vi "main.vi"() -> ()   [LabVIEW 2018]
uses:
  <vilib>/NI/Modbus Library/API/Wrapper/Create TCP Slave.vi
  <vilib>/NI/Modbus Library/API/Slave/Modbus Slave.lvclass
  <vilib>/NI/Modbus Library/API/Wrapper/API Main.lvlib
panel:
  out "TCP Connection Count":u32
  in  "擦除曲线":bool
  in  "PC启动信号":bool
  in  "PC就绪":bool
  out "远程/本地控制布尔":bool
  out "XY图":cluster{i32[], sgl[]}[](graph)
  in  "远程/本地控制":bool
  out "远程/本地控制标题":string="远程/本地"
  out "当前档位":string="当前档位"
  in  "档位目标内容":string
  out "PCTOUTAC的当前档位":string="PCTOUTAC的当前档位"
  out "档位目标内容远程":string
  in  "档位目标内容本地":string
  out "档位目标":string="配方编号"
  out "UTACTOPC的目标档位":string="UTACTOPC的配方编号"
  in  "中英文":string(combo)
  in  "编辑设定参数":bool
  in  "编辑配方":bool
  in  "退出":bool
  out "设置":string="设置"
  in  "PC换挡不成功":bool
  in  "PC换挡到位":bool
  in  "PC正在换挡":bool
  in  "PC急停":bool
  in  "PC学习":bool
  in  "PC故障":bool
  in  "PC运行/停机":bool
  out "PCOUTAC的DI信号":string="PCTOUTAC的DI信号"
  in  "UTAC复位到原点":bool
  in  "UTAC故障复位":bool
  in  "UTAC急停":bool
  in  "UTAC故障":bool
  in  "UTAC运行/停机":bool
  out "UTACTOPC的DO信号":string="UTACTOPC的DO信号"
  in  "设置":bool
  in  "总测试次数文本":string
  in  "动作数量文本":string
  in  "备注文本":string
  in  "样品编号文本":string
  in  "零件编号文本":string
  in  "零件名称文本":string
  in  "项目编号文本":string
  out "总测试次数":string="总测试次数"
  out "动作数量":string="动作数量"
  out "备注":string="备注"
  out "样品编号":string="样品编号"
  out "零件编号":string="零件编号"
  out "零件名称":string="零件名称"
  out "项目编号":string="项目编号"
  out "项目信息":string="项目信息"
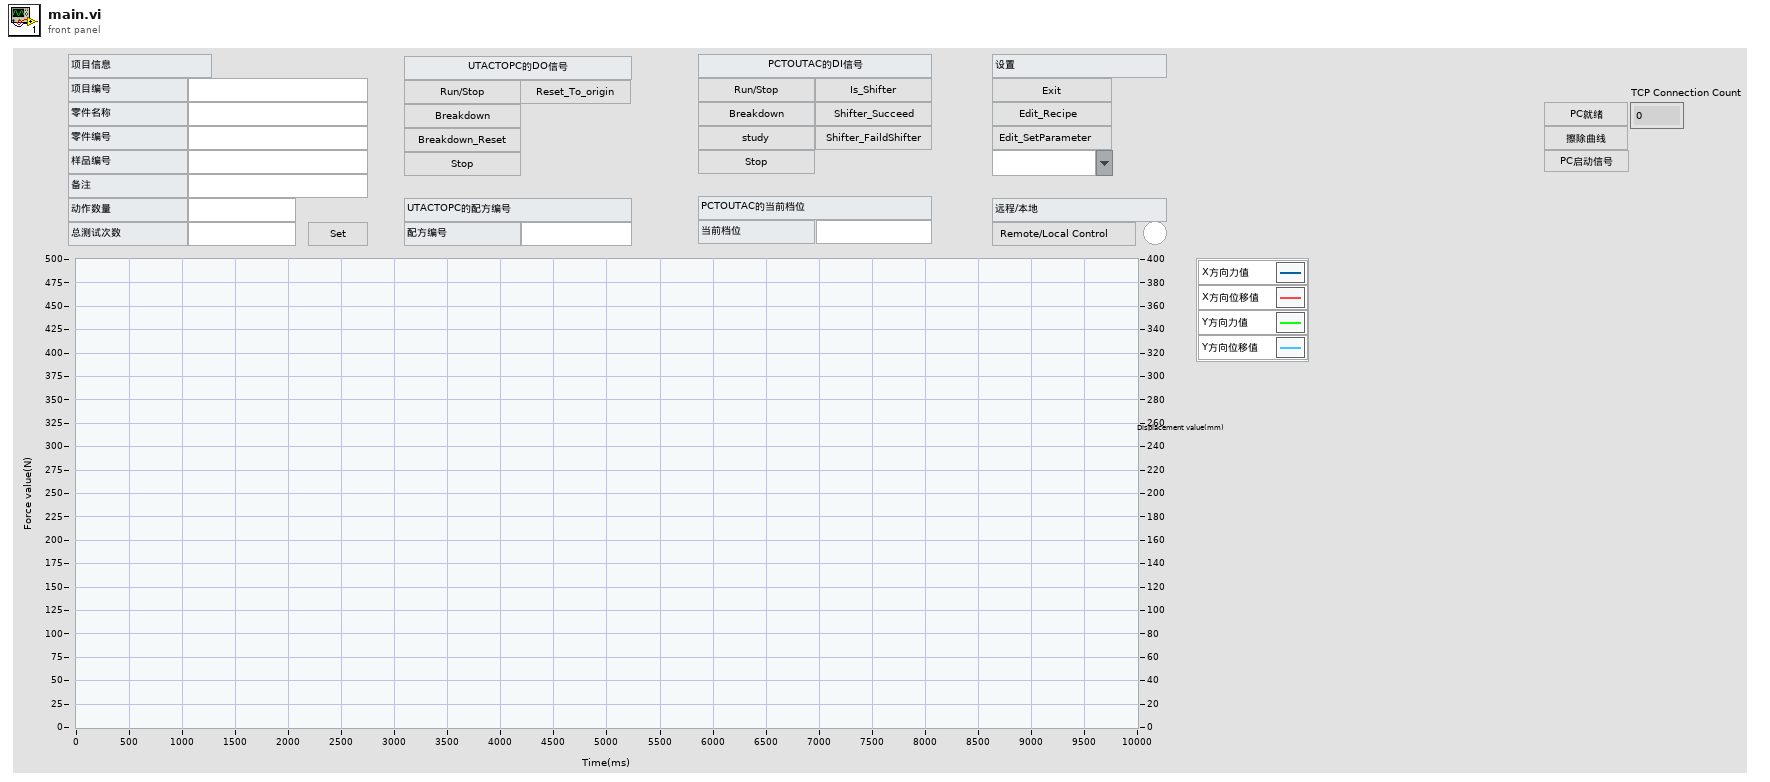
[diagram p1: front panel]
types:
  T1 = cluster{"主站IP":u32, "组号":u8, "帧号":u16, "时间戳":u64}
  T2 = cluster{"X方向力值":sgl, "Y方向力值":sgl, "X方向位移值":sgl, "Y方向位移值":sgl}
  T3 = cluster{"挡位N1所在序号":sgl, "挡位1所在序号":sgl, "挡位N1所在序号":sgl, "挡位2所在序号":sgl, "挡位N1所在序号":sgl, " 挡位N2所在序号":sgl, "挡位3所在序号":sgl, "挡位N2所在序号":sgl, "挡位4所在序号":sgl, " 挡位N2所在序号":sgl, "挡位N3所在序号":sgl, "挡位5所在序号":sgl, "挡位N3所在序号":sgl, "挡位6所在序号":sgl, "挡位N3所在序号":sgl, "挡位N4所在序号":sgl, " 挡位7所在序号":sgl, " 挡位N4所在序号":sgl, "挡位8所在序号":sgl, "挡位N4所在序号":sgl, " 挡位N5所在序号":sgl, "挡位9所在序号":sgl, "挡位N5所在序号":sgl, " 挡位10所在序号":sgl}
  T4 = cluster{"就绪":bool, "运行/停机":bool, "故障":bool, "学习":bool, "急停":bool, "正在换挡":bool, "换挡到位":bool, "换挡不成功":bool, "备用1":bool, "保存开始":bool, "等待下发任务":bool, "允许读取配方":bool, "开始采集数据":bool, "时间ON/OFF":bool, " 收到启动信号":bool, "结束采集信号":bool, "读配方参数ON/OFF":bool, "允许下发配方参数":bool}
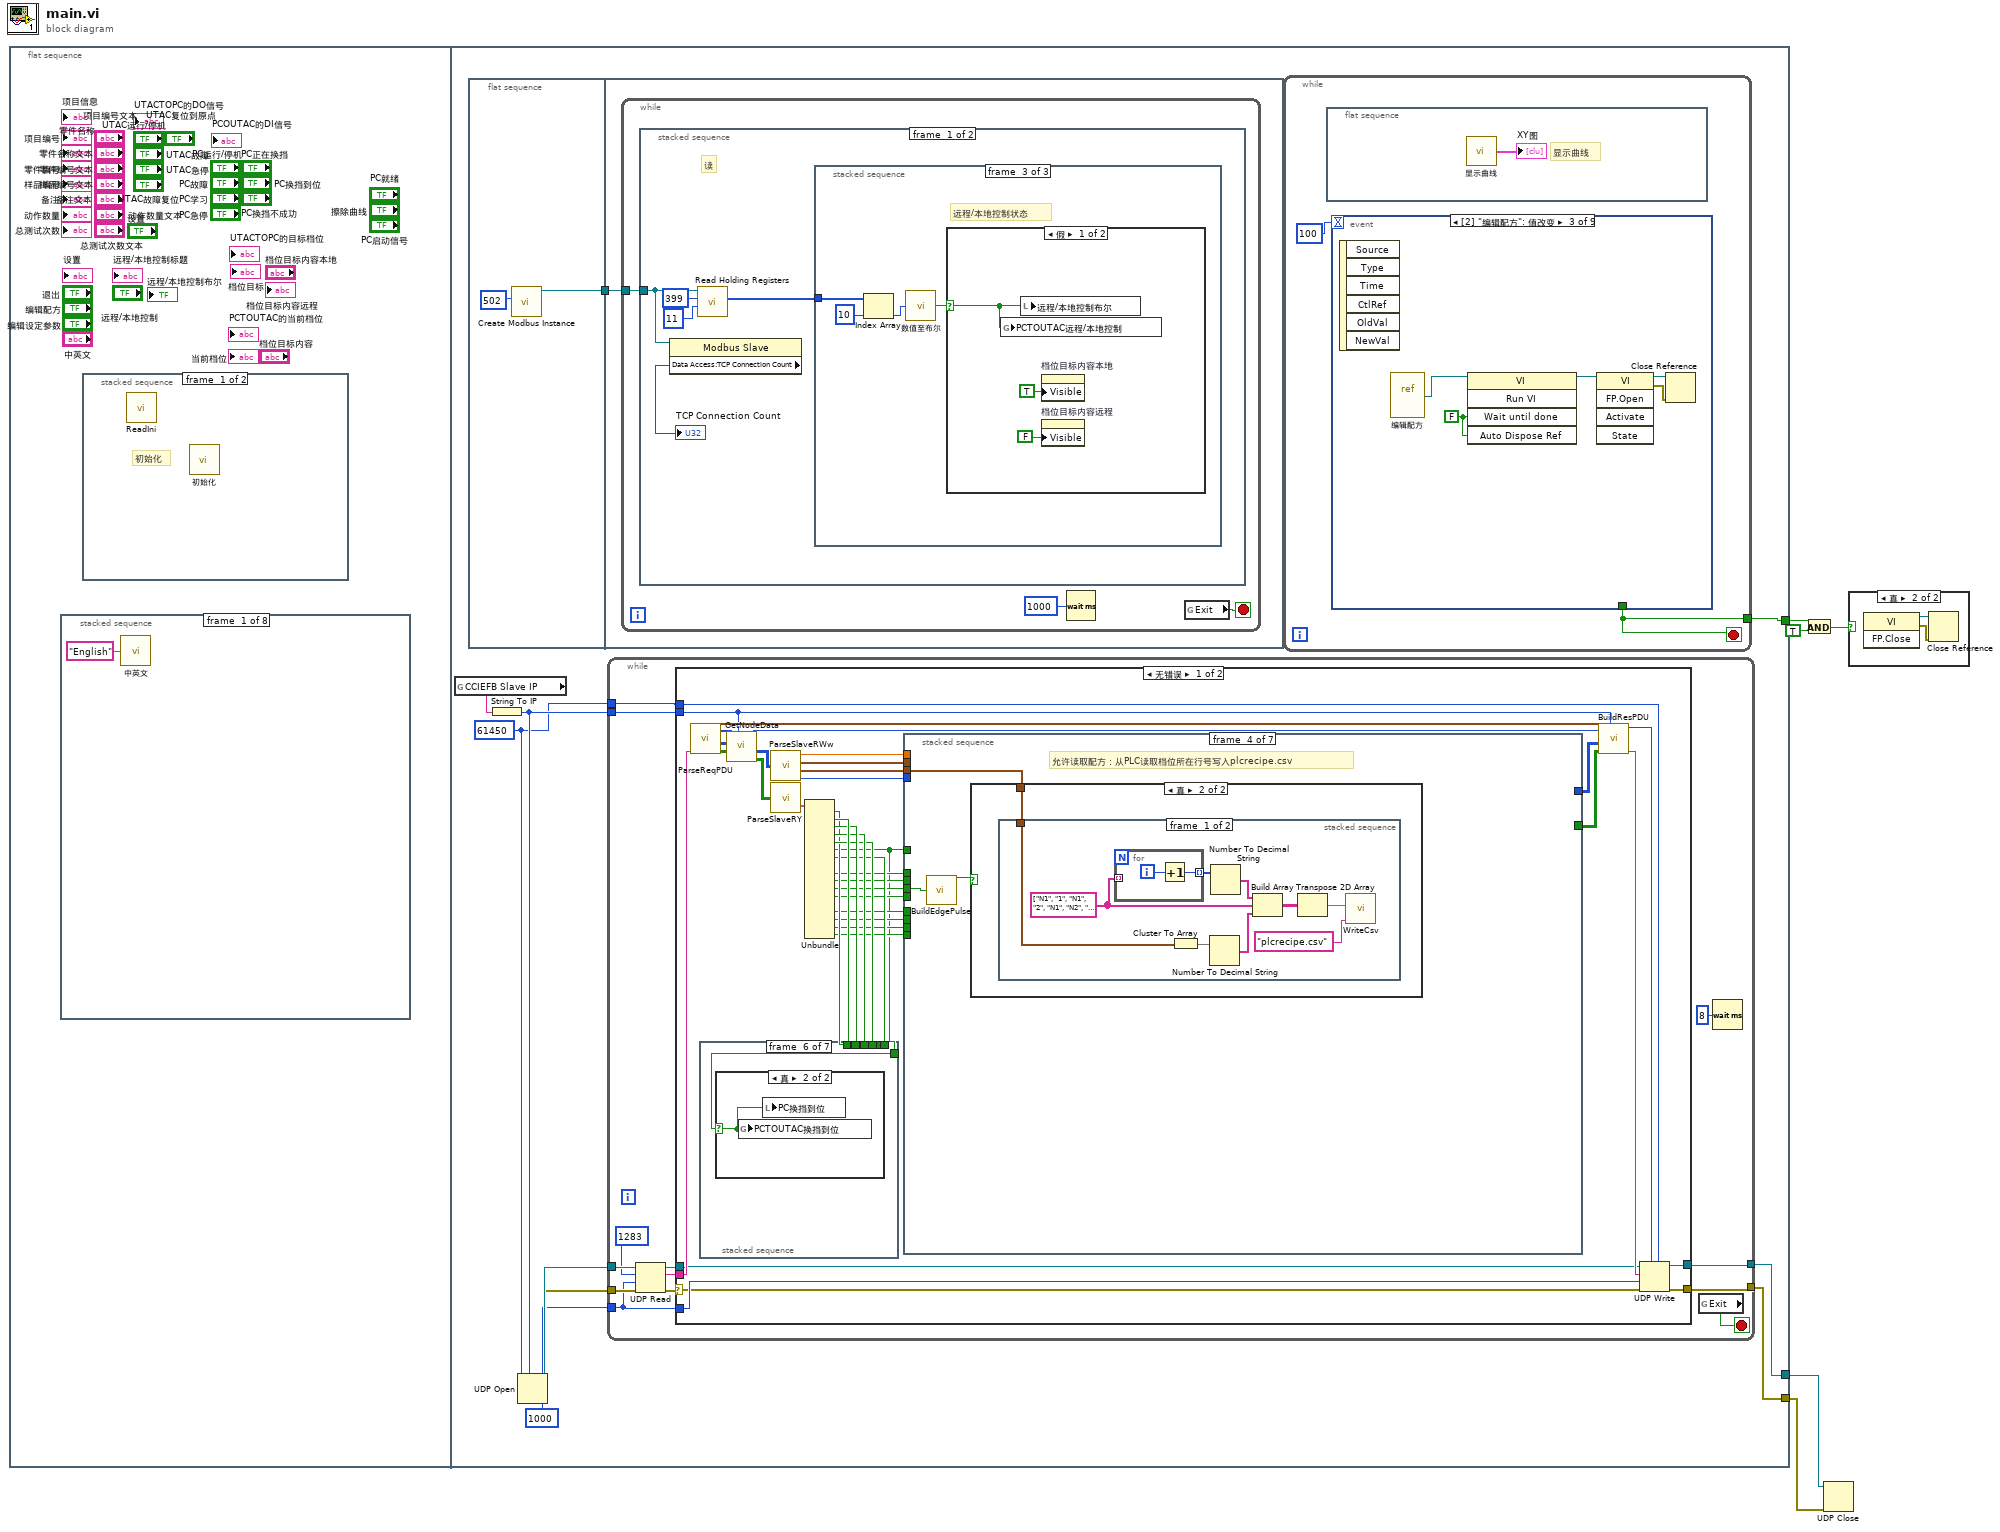
[diagram p0: block diagram]
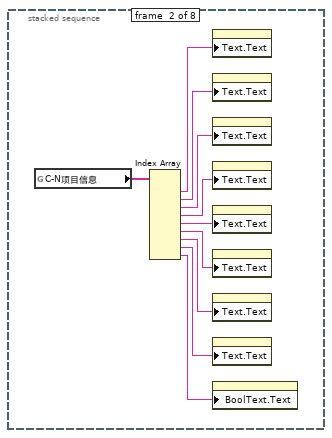
[diagram p3: hidden frame]
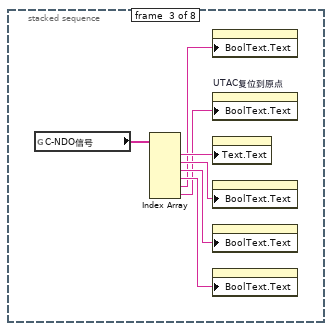
[diagram p4: hidden frame]
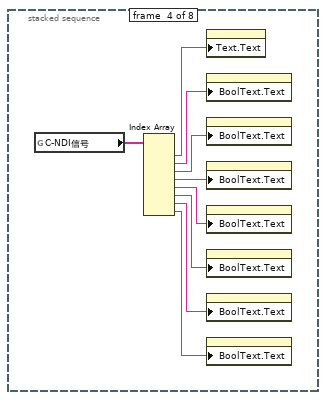
[diagram p5: hidden frame]
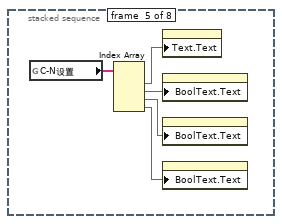
[diagram p6: hidden frame]
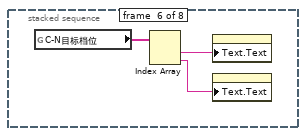
[diagram p7: hidden frame]
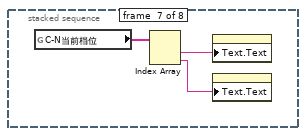
[diagram p8: hidden frame]
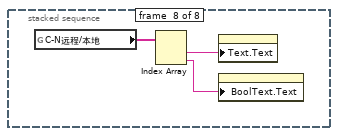
[diagram p9: hidden frame]
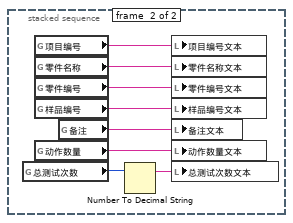
[diagram p10: hidden frame]
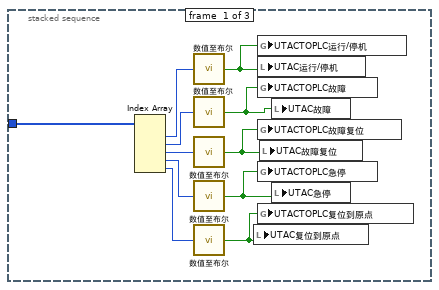
[diagram p11: hidden frame]
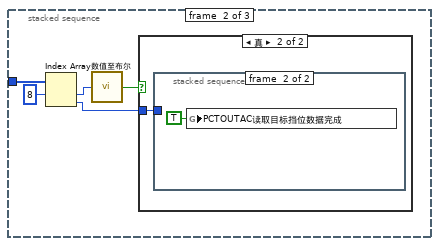
[diagram p12: hidden frame]
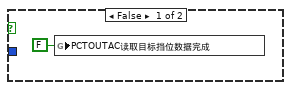
[diagram p13: hidden frame]
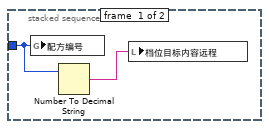
[diagram p14: hidden frame]
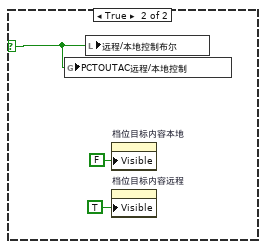
[diagram p15: hidden frame]
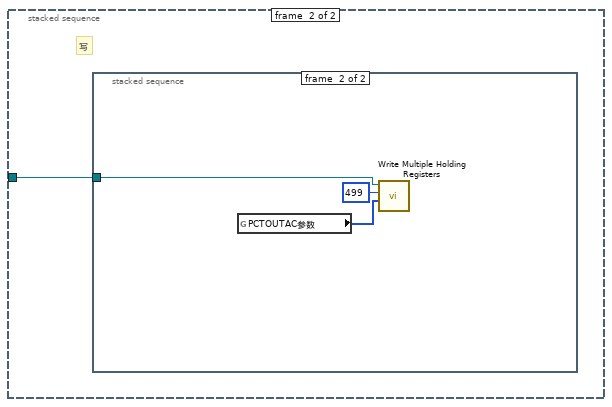
[diagram p16: hidden frame]
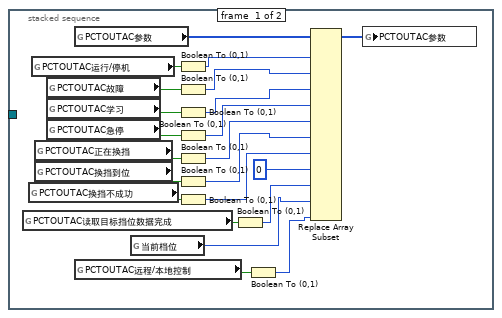
[diagram p17: hidden frame]
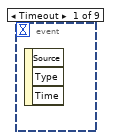
[diagram p18: hidden frame]
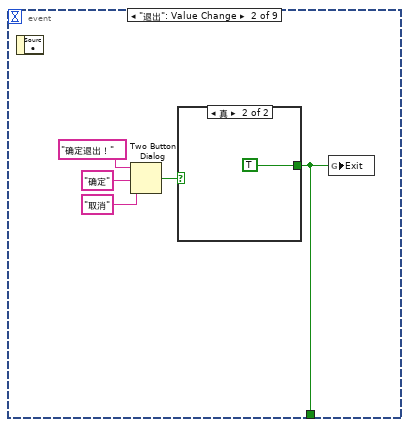
[diagram p19: hidden frame]
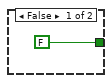
[diagram p20: hidden frame]
diagram:
  n1 = flat-sequence {
    tunnel: [w62] -> w5
    tunnel: [w61] -> w4
    tunnel: [w56] -> w3
    frame #0 {
      n2 = stacked-sequence {
        frame #0 {
          n3 = call "中英文.vi"("中英文"="English") -> ()  [unwired: 2 in]
        }
        frame #1 {
          n4 = global read "全局 1.vi" "C-N项目信息"() -> (w16:string[])
          n5 = Index Array(array=w16) -> (element #1=w15:string, element #2=w14:string, element #3=w13:string, element #4=w12:string, element #5=w11:string, element #6=w10:string, element #7=w9:string, element #8=w8:string, element #9=w7:string)  [unwired: 9 in]
          n6 = property on="项目信息" class="Str"("Text.Text"=w15) -> ()  [unwired: 2 in, 2 out]
          n7 = property on="项目编号" class="Str"("Text.Text"=w14) -> ()  [unwired: 2 in, 2 out]
          n8 = property on="零件名称" class="Str"("Text.Text"=w13) -> ()  [unwired: 2 in, 2 out]
          n9 = property on="零件编号" class="Str"("Text.Text"=w12) -> ()  [unwired: 2 in, 2 out]
          n10 = property on="样品编号" class="Str"("Text.Text"=w11) -> ()  [unwired: 2 in, 2 out]
          n11 = property on="备注" class="Str"("Text.Text"=w10) -> ()  [unwired: 2 in, 2 out]
          n12 = property on="动作数量" class="Str"("Text.Text"=w9) -> ()  [unwired: 2 in, 2 out]
          n13 = property on="总测试次数" class="Str"("Text.Text"=w8) -> ()  [unwired: 2 in, 2 out]
          n14 = property on="设置" class="Bool"("BoolText.Text"=w7) -> ()  [unwired: 2 in, 2 out]
        }
        frame #2 {
          n15 = global read "全局 1.vi" "C-NDO信号"() -> (w23:string[])
          n16 = Index Array(array=w23) -> (element #1=w22:string, element #2=w21:string, element #3=w20:string, element #4=w19:string, element #5=w18:string, element #6=w17:string)  [unwired: 6 in]
          n17 = property on="UTAC急停" class="Bool (严格)"("BoolText.Text"=w18) -> ()  [unwired: 2 in, 2 out]
          n18 = property on="UTAC复位到原点" class="Bool (严格)"("BoolText.Text"=w17) -> ()  [unwired: 2 in, 2 out]
          n19 = property on="UTACTOPC的DO信号" class="Str"("Text.Text"=w22) -> ()  [unwired: 2 in, 2 out]
          n20 = property on="UTAC运行/停机" class="Bool (严格)"("BoolText.Text"=w21) -> ()  [unwired: 2 in, 2 out]
          n21 = property on="UTAC故障" class="Bool (严格)"("BoolText.Text"=w20) -> ()  [unwired: 2 in, 2 out]
          n22 = property on="UTAC故障复位" class="Bool (严格)"("BoolText.Text"=w19) -> ()  [unwired: 2 in, 2 out]
        }
        frame #3 {
          n23 = global read "全局 1.vi" "C-NDI信号"() -> (w32:string[])
          n24 = Index Array(array=w32) -> (element #1=w31:string, element #2=w30:string, element #3=w29:string, element #4=w28:string, element #5=w27:string, element #6=w26:string, element #7=w25:string, element #8=w24:string)  [unwired: 8 in]
          n25 = property on="PCOUTAC的DI信号" class="Str"("Text.Text"=w31) -> ()  [unwired: 2 in, 2 out]
          n26 = property on="PC运行/停机" class="Bool (严格)"("BoolText.Text"=w30) -> ()  [unwired: 2 in, 2 out]
          n27 = property on="PC故障" class="Bool (严格)"("BoolText.Text"=w29) -> ()  [unwired: 2 in, 2 out]
          n28 = property on="PC学习" class="Bool (严格)"("BoolText.Text"=w28) -> ()  [unwired: 2 in, 2 out]
          n29 = property on="PC急停" class="Bool (严格)"("BoolText.Text"=w27) -> ()  [unwired: 2 in, 2 out]
          n30 = property on="PC正在换挡" class="Bool (严格)"("BoolText.Text"=w26) -> ()  [unwired: 2 in, 2 out]
          n31 = property on="PC换挡到位" class="Bool (严格)"("BoolText.Text"=w25) -> ()  [unwired: 2 in, 2 out]
          n32 = property on="PC换挡不成功" class="Bool (严格)"("BoolText.Text"=w24) -> ()  [unwired: 2 in, 2 out]
        }
        frame #4 {
          n33 = global read "全局 1.vi" "C-N设置"() -> (w37:string[])
          n34 = Index Array(array=w37) -> (element #1=w36:string, element #2=w35:string, element #3=w34:string, element #4=w33:string)  [unwired: 4 in]
          n35 = property on="设置" class="Str"("Text.Text"=w36) -> ()  [unwired: 2 in, 2 out]
          n36 = property on="退出" class="Bool"("BoolText.Text"=w35) -> ()  [unwired: 2 in, 2 out]
          n37 = property on="编辑配方" class="Bool"("BoolText.Text"=w34) -> ()  [unwired: 2 in, 2 out]
          n38 = property on="编辑设定参数" class="Bool"("BoolText.Text"=w33) -> ()  [unwired: 2 in, 2 out]
        }
        frame #5 {
          n39 = global read "全局 1.vi" "C-N目标档位"() -> (w40:string[])
          n40 = Index Array(array=w40) -> (element #1=w39:string, element #2=w38:string)  [unwired: 2 in]
          n41 = property on="UTACTOPC的目标档位" class="Str"("Text.Text"=w39) -> ()  [unwired: 2 in, 2 out]
          n42 = property on="档位目标" class="Str"("Text.Text"=w38) -> ()  [unwired: 2 in, 2 out]
        }
        frame #6 {
          n43 = global read "全局 1.vi" "C-N当前档位"() -> (w43:string[])
          n44 = Index Array(array=w43) -> (element #1=w42:string, element #2=w41:string)  [unwired: 2 in]
          n45 = property on="PCTOUTAC的当前档位" class="Str"("Text.Text"=w42) -> ()  [unwired: 2 in, 2 out]
          n46 = property on="当前档位" class="Str"("Text.Text"=w41) -> ()  [unwired: 2 in, 2 out]
        }
        frame #7 {
          n47 = global read "全局 1.vi" "C-N远程/本地"() -> (w46:string[])
          n48 = Index Array(array=w46) -> (element #1=w45:string, element #2=w44:string)  [unwired: 2 in]
          n49 = property on="远程/本地控制标题" class="Str"("Text.Text"=w45) -> ()  [unwired: 2 in, 2 out]
          n50 = property on="远程/本地控制" class="Bool (严格)"("BoolText.Text"=w44) -> ()  [unwired: 2 in, 2 out]
        }
      }
      n51 = stacked-sequence {
        frame #0 {
          # "初始化"
          n52 = call "ReadIni.vi"() -> ()  [unwired: 2 in]
          n53 = call "初始化.vi"() -> ()  [unwired: 12 in]
        }
        frame #1 {
          n54 = global read "全局 1.vi" "总测试次数"() -> (w54:i16)
          n55 = global read "全局 1.vi" "项目编号"() -> (w52:string)
          n56 = global read "全局 1.vi" "零件名称"() -> (w51:string)
          n57 = global read "全局 1.vi" "零件编号"() -> (w50:string)
          n58 = global read "全局 1.vi" "样品编号"() -> (w49:string)
          n59 = global read "全局 1.vi" "动作数量"() -> (w47:string)
          n60 = global read "全局 1.vi" "备注"() -> (w48:string)
          n61 = Number To Decimal String(number=w54) -> (decimal integer string=w53:string)  [unwired: 1 in]
          n62 = local write "项目编号文本"(w52) -> ()
          n63 = local write "零件名称文本"(w51) -> ()
          n64 = local write "零件编号文本"(w50) -> ()
          n65 = local write "样品编号文本"(w49) -> ()
          n66 = local write "备注文本"(w48) -> ()
          n67 = local write "动作数量文本"(w47) -> ()
          n68 = local write "总测试次数文本"(w53) -> ()
        }
      }
    }
    frame #1 {
      w57 = u16 61450
      n69 = global read "全局 1.vi" "CCIEFB Slave IP"() -> (w60:string)
      n70 = flat-sequence {
        tunnel: [w65] -> w55
        tunnel: w55 -> [w67]
        frame #0 {
          n71 = call-poly <vilib>:"Create Modbus Instance.vi"("port (502)"=u16 502) -> ("TCP slave instance"=w65:refnum<class "Modbus Slave.lvclass">)  [unwired: 9 in, 1 out]
        }
        frame #1 {
          n72 = while {
            tunnel: w67 -> [w69]
            stop <- w70 stop-if-true
            n73 = stacked-sequence {
              tunnel: w69 -> [w72 w107]
              frame #0 {
                # "读"
                n74 = property class="Modbus Slave"(reference=w72) -> ("Data Access:TCP Connection Count"=→"TCP Connection Count":u32)  [unwired: 1 in, 2 out]
                n75 = call-dynamic "Read Holding Registers.vi"("number of inputs"=u16 11, "starting address"=u16 399, "Modbus slave in"=w72) -> ("register values"=w73:u16[])  [unwired: 6 in, 2 out]
                n76 = stacked-sequence {
                  tunnel: w73 -> [w86 w91 w100]
                  frame #0 {
                    n77 = Index Array(array=w86) -> (element #1=w85:u16, element #2=w84:u16, element #3=w83:u16, element #4=w82:u16, element #5=w81:u16)  [unwired: 5 in]
                    n78 = call "数值至布尔.vi"("数值"=w85) -> ("布尔"=w80:bool)
                    n79 = call "数值至布尔.vi"("数值"=w84) -> ("布尔"=w79:bool)
                    n80 = call "数值至布尔.vi"("数值"=w83) -> ("布尔"=w78:bool)
                    n81 = call "数值至布尔.vi"("数值"=w82) -> ("布尔"=w77:bool)
                    n82 = call "数值至布尔.vi"("数值"=w81) -> ("布尔"=w76:bool)
                    n83 = local write "UTAC复位到原点"(w76) -> ()
                    n84 = global write "全局 1.vi" "UTACTOPLC运行/停机"(w80) -> ()
                    n85 = local write "UTAC运行/停机"(w80) -> ()
                    n86 = global write "全局 1.vi" "UTACTOPLC故障"(w79) -> ()
                    n87 = global write "全局 1.vi" "UTACTOPLC故障复位"(w78) -> ()
                    n88 = global write "全局 1.vi" "UTACTOPLC急停"(w77) -> ()
                    n89 = global write "全局 1.vi" "UTACTOPLC复位到原点"(w76) -> ()
                    n90 = local write "UTAC故障复位"(w78) -> ()
                    n91 = local write "UTAC故障"(w79) -> ()
                    n92 = local write "UTAC急停"(w77) -> ()
                  }
                  frame #1 {
                    n93 = Index Array(array=w91, index #1=8 ("索引")) -> (element #1=w89:u16, element #2=w87:u16)  [unwired: 1 in]
                    n94 = call "数值至布尔.vi"("数值"=w89) -> ("布尔"=w88:bool)
                    n95 = case shown="真" w88 {
                      tunnel: w87 -> [_ w93]
                      frame False {
                        n96 = global write "全局 1.vi" "PCTOUTAC读取目标挡位数据完成"(FALSE ("PCTOUTAC读取目标挡位数据完成")) -> ()
                      }
                      frame True {
                        n97 = stacked-sequence {
                          tunnel: w93 -> [w95 _]
                          frame #0 {
                            n98 = global write "全局 1.vi" "配方编号"(w95) -> ()
                            n99 = Number To Decimal String(number=w95) -> (decimal integer string=w94:string)  [unwired: 1 in]
                            n100 = local write "档位目标内容远程"(w94) -> ()
                          }
                          frame #1 {
                            n101 = global write "全局 1.vi" "PCTOUTAC读取目标挡位数据完成"(TRUE ("PCTOUTAC读取目标挡位数据完成")) -> ()
                          }
                        }
                      }
                    }
                  }
                  frame #2 {
                    # "远程/本地控制状态"
                    n102 = Index Array(array=w100, index=10 ("索引")) -> (element=w98:u16)
                    n103 = call "数值至布尔.vi"("数值"=w98) -> ("布尔"=w97:bool)
                    n104 = case shown="假" w97 {
                      selector: w97 -> [w103 w106]
                      frame False {
                        n105 = global write "全局 1.vi" "PCTOUTAC远程/本地控制"(w103) -> ()
                        n106 = local write "远程/本地控制布尔"(w103) -> ()
                        n107 = property on="档位目标内容本地" class="Str"("Visible"=TRUE ("可见")) -> ()  [unwired: 2 in, 2 out]
                        n108 = property on="档位目标内容远程" class="Str"("Visible"=FALSE ("可见")) -> ()  [unwired: 2 in, 2 out]
                      }
                      frame True {
                        n109 = global write "全局 1.vi" "PCTOUTAC远程/本地控制"(w106) -> ()
                        n110 = local write "远程/本地控制布尔"(w106) -> ()
                        n111 = property on="档位目标内容本地" class="Str"("Visible"=FALSE ("可见")) -> ()  [unwired: 2 in, 2 out]
                        n112 = property on="档位目标内容远程" class="Str"("Visible"=TRUE ("可见")) -> ()  [unwired: 2 in, 2 out]
                      }
                    }
                  }
                }
              }
              frame #1 {
                # "写"
                n113 = stacked-sequence {
                  tunnel: w107 -> [_ w132]
                  frame #0 {
                    n114 = global read "全局 1.vi" "PCTOUTAC读取目标挡位数据完成"() -> (w112:bool)
                    n115 = global read "全局 1.vi" "PCTOUTAC换挡不成功"() -> (w123:bool)
                    n116 = global read "全局 1.vi" "PCTOUTAC运行/停机"() -> (w129:bool)
                    n117 = global read "全局 1.vi" "PCTOUTAC正在换挡"() -> (w125:bool)
                    n118 = global read "全局 1.vi" "PCTOUTAC换挡到位"() -> (w124:bool)
                    n119 = global read "全局 1.vi" "PCTOUTAC故障"() -> (w128:bool)
                    n120 = global read "全局 1.vi" "PCTOUTAC学习"() -> (w127:bool)
                    n121 = global read "全局 1.vi" "PCTOUTAC急停"() -> (w126:bool)
                    n122 = global read "全局 1.vi" "PCTOUTAC参数"() -> (w122:i16[])
                    n123 = global read "全局 1.vi" "PCTOUTAC远程/本地控制"() -> (w109:bool)
                    n124 = global read "全局 1.vi" "当前档位"() -> (w110:u16)
                    n125 = Boolean To (0,1)(Boolean=w129) -> (0, 1=w121:i16)
                    n126 = Boolean To (0,1)(Boolean=w128) -> (0, 1=w119:i16)
                    n127 = Boolean To (0,1)(Boolean=w127) -> (0, 1=w118:i16)
                    n128 = Boolean To (0,1)(Boolean=w126) -> (0, 1=w117:i16)
                    n129 = Boolean To (0,1)(Boolean=w125) -> (0, 1=w116:i16)
                    n130 = Boolean To (0,1)(Boolean=w124) -> (0, 1=w115:i16)
                    n131 = Boolean To (0,1)(Boolean=w123) -> (0, 1=w114:i16)
                    n132 = Boolean To (0,1)(Boolean=w112) -> (0, 1=w111:i16)
                    n133 = Boolean To (0,1)(Boolean=w109) -> (0, 1=w108:i16)
                    n134 = Replace Array Subset(array=w122, new element #1=w121, new element #2=w119, new element #3=w118, new element #4=w117, new element #5=w116, new element #6=w115, new element #7=w114, new element #8=i16 0 ("新元素/子数组"), new element #9=w111, new element #10=w110, new element #11=w108) -> (w120:i16[])  [unwired: 11 in]
                    n135 = global write "全局 1.vi" "PCTOUTAC参数"(w120) -> ()
                  }
                  frame #1 {
                    n136 = global read "全局 1.vi" "PCTOUTAC参数"() -> (w130:i16[])
                    n137 = call-dynamic "Write Multiple Holding Registers.vi"("registers to write"=w130, "starting address"=u16 499, "Modbus slave in"=w132) -> ()  [unwired: 7 in, 2 out]
                  }
                }
              }
            }
            n138 = Wait (ms)(milliseconds to wait=u32 1000 ("等待时间（毫秒）")) -> ()  [unwired: 1 out]
            n139 = global read "全局 1.vi" "Exit"() -> (w70:bool)
          }
        }
      }
      n140 = String To IP(1:w60) -> (0:w58:u32)
      n141 = UDP Open(7:w58, 11:w57) -> (port=w64:refnum<k16>, 0:w63:errorcluster)  [unwired: 3 in, 1 out]
      n142 = while {
        tunnel: w64 -> [w219]
        tunnel: w63 -> [w218]
        tunnel: [w211] -> w62
        tunnel: [w210] -> w61
        tunnel: 1000 -> [w209]
        tunnel: w58 -> [w212]
        tunnel: w57 -> [w208]
        stop <- w217 stop-if-true
        n143 = UDP Read(connection ID=w219, max size (548)=1283 ("最大值(548)"), timeout ms (25000)=w209, 8:w218) -> (data out=w214:string, error out=w215:errorcluster, 3:w213:refnum<k16>)  [unwired: 2 out]
        n144 = case shown="无错误" w215 {
          selector: w215 -> [w246 w363]
          tunnel: w214 -> [w258 _]
          tunnel: w213 -> [w248 w361]
          tunnel: [w251 w362] -> w210
          tunnel: [w250 w361] -> w211
          tunnel: w212 -> [w243 _]
          tunnel: w209 -> [w247 _]
          tunnel: w208 -> [w242 _]
          frame No Error {
            n145 = call "ParseReqPDU.vi"("数据in"=w258) -> ("All RY"=w255:bool[][], "All RWw"=w256:u16[][], "从站IP组"=w257:u32[], "主站信息"=w252:T1)  [unwired: 7 in]
            n146 = call "GetNodeData.vi"("指定从站IP"=w243, "All RY in"=w255, "All RWw in"=w256, "从站IP组"=w257) -> ("Node RY"=w253:bool[][], "Node RWw"=w254:u16[][], "占用站数"=w244:i32)  [unwired: 5 in]
            n147 = call "ParseSlaveRWw.vi"("Node RWw"=w254) -> ("当前档位"=w239:sgl, "PLC采集值"=w238:T2, "PLC档位序号"=w237:T3, "行号"=w236:i32)
            n148 = call "ParseSlaveRY.vi"("RY"=w253) -> ("PLC状态"=w235:T4)  [unwired: 1 in]
            n149 = Unbundle(w235) -> ("运行/停机"=w230:bool, "故障"=w234:bool, "学习"=w233:bool, "急停"=w232:bool, "正在换挡"=w231:bool, "换挡到位"=w220:bool, "换挡不成功"=w229:bool, "保存开始"=w228:bool, "等待下发任务"=w227:bool, "允许读取配方"=w221:bool, "开始采集数据"=w226:bool, "收到启动信号"=w224:bool, "结束采集信号"=w225:bool, "读配方参数ON/OFF"=w223:bool, "允许下发配方参数"=w222:bool)  [unwired: 3 out]
            n150 = stacked-sequence {
              tunnel: w230 -> [w259 _ _ _ _ _ _]
              tunnel: w234 -> [_ w261 _ _ _ _ _]
              tunnel: w233 -> [_ _ w263 _ _ _ _]
              tunnel: w232 -> [_ _ _ w265 _ _ _]
              tunnel: w231 -> [_ _ _ _ w267 _ w271]
              tunnel: w220 -> [_ _ _ _ _ w269 _]
              tunnel: w229 -> [_ _ _ _ _ _ _]
              frame #0 {
                n151 = case shown="真" w259 {
                  selector: w259 -> [_ w260]
                  frame False {
                  }
                  frame True {
                    n152 = global write "全局 1.vi" "PCTOUTAC运行/停机"(w260) -> ()
                    n153 = local write "PC运行/停机"(w260) -> ()
                  }
                }
              }
              frame #1 {
                n154 = case shown="真" w261 {
                  selector: w261 -> [_ w262]
                  frame False {
                  }
                  frame True {
                    n155 = global write "全局 1.vi" "PCTOUTAC故障"(w262) -> ()
                    n156 = local write "PC故障"(w262) -> ()
                  }
                }
              }
              frame #2 {
                n157 = case shown="真" w263 {
                  selector: w263 -> [_ w264]
                  frame False {
                  }
                  frame True {
                    n158 = global write "全局 1.vi" "PCTOUTAC学习"(w264) -> ()
                    n159 = local write "PC学习"(w264) -> ()
                  }
                }
              }
              frame #3 {
                n160 = case shown="真" w265 {
                  selector: w265 -> [_ w266]
                  frame False {
                  }
                  frame True {
                    n161 = global write "全局 1.vi" "PCTOUTAC急停"(w266) -> ()
                    n162 = local write "PC急停"(w266) -> ()
                  }
                }
              }
              frame #4 {
                n163 = case shown="真" w267 {
                  selector: w267 -> [_ w268]
                  frame False {
                  }
                  frame True {
                    n164 = global write "全局 1.vi" "PCTOUTAC正在换挡"(w268) -> ()
                    n165 = local write "PC正在换挡"(w268) -> ()
                  }
                }
              }
              frame #5 {
                n166 = case shown="真" w269 {
                  selector: w269 -> [_ w270]
                  frame False {
                  }
                  frame True {
                    n167 = global write "全局 1.vi" "PCTOUTAC换挡到位"(w270) -> ()
                    n168 = local write "PC换挡到位"(w270) -> ()
                  }
                }
              }
              frame #6 {
                n169 = case shown="真" w271 {
                  selector: w271 -> [_ w272]
                  frame False {
                  }
                  frame True {
                    n170 = global write "全局 1.vi" "PCTOUTAC正在换挡"(w272) -> ()
                    n171 = local write "PC换挡不成功"(w272) -> ()
                  }
                }
              }
            }
            n172 = stacked-sequence {
              tunnel: [_ _ _ _ _ _ w360] -> w241
              tunnel: [_ _ _ _ _ _ w359] -> w240
              tunnel: w239 -> [_ _ _ _ w321 _ _]
              tunnel: w238 -> [_ _ _ _ w322 _ _]
              tunnel: w237 -> [_ _ _ w304 _ _ _]
              tunnel: w236 -> [_ _ _ _ _ w341 _]
              tunnel: w228 -> [w274 w292 _ _ _ _ _]
              tunnel: w227 -> [w273 _ w295 _ _ _ _]
              tunnel: w221 -> [w278 _ _ w305 _ _ _]
              tunnel: w226 -> [_ _ _ _ w324 _ _]
              tunnel: w225 -> [_ _ _ _ _ _ _]
              tunnel: w224 -> [w277 _ _ _ w323 _ _]
              tunnel: w223 -> [w275 _ _ _ _ w343 _]
              tunnel: w222 -> [w276 _ _ _ _ w342 _]
              tunnel: w220 -> [_ _ _ _ w320 _ _]
              frame #0 {
                # "收到启动信号"
                n173 = stacked-sequence {
                  tunnel: w278 -> [_ _ w283 _ _ _]
                  tunnel: w277 -> [_ _ _ w285 _ _]
                  tunnel: w276 -> [_ _ _ _ w287 _]
                  tunnel: w275 -> [_ _ _ _ _ w289]
                  tunnel: w274 -> [w279 _ _ _ _ _]
                  tunnel: w273 -> [_ w281 _ _ _ _]
                  frame #0 {
                    n174 = case shown="假" w279 {
                      frame False {
                        n175 = global write "全局 1.vi" "PCTOPLC保存完成"(FALSE ("PCTOPLC保存完成")) -> ()
                      }
                      frame True {
                      }
                    }
                  }
                  frame #1 {
                    n176 = case shown="假" w281 {
                      frame False {
                        n177 = global write "全局 1.vi" "PCTOPLC下发任务完成"(FALSE ("PCTOPLC保存完成")) -> ()
                      }
                      frame True {
                      }
                    }
                  }
                  frame #2 {
                    n178 = case shown="假" w283 {
                      frame False {
                        n179 = global write "全局 1.vi" "PCTOPLC读取配方完成"(FALSE ("PCTOUTAC换挡到位")) -> ()
                      }
                      frame True {
                      }
                    }
                  }
                  frame #3 {
                    n180 = case shown="假" w285 {
                      frame False {
                        n181 = global write "全局 1.vi" "PCTOPLC发送启动信号"(FALSE ("PCTOUTAC换挡到位")) -> ()
                      }
                      frame True {
                      }
                    }
                  }
                  frame #4 {
                    n182 = case shown="假" w287 {
                      frame False {
                        n183 = global write "全局 1.vi" "PCTOPLC下发配方参数完成"(FALSE ("PCTOPLC下发配方参数完成")) -> ()
                      }
                      frame True {
                      }
                    }
                  }
                  frame #5 {
                    n184 = case shown="假" w289 {
                      frame False {
                        n185 = global write "全局 1.vi" "PCTOPLC读配方结束"(FALSE ("PCTOPLC下发配方参数完成")) -> ()
                      }
                      frame True {
                      }
                    }
                  }
                }
              }
              frame #1 {
                # "保存"
                n186 = call "BuildEdgePulse.vi"("输入"=w292) -> ("上升沿"=w291:bool)  [unwired: 2 in, 2 out]
                n187 = case shown="真" w291 {
                  frame False {
                  }
                  frame True {
                    n188 = stacked-sequence {
                      frame #0 {
                        n189 = call "保存模版.vi"() -> ()  [unwired: 12 in]
                      }
                      frame #1 {
                        n190 = global write "全局 1.vi" "PCTOPLC保存完成"(TRUE ("PCTOPLC保存完成")) -> ()
                      }
                    }
                  }
                }
              }
              frame #2 {
                # "等待下发任务"
                n191 = call "BuildEdgePulse.vi"("输入"=w295) -> ("上升沿"=w294:bool)  [unwired: 2 in, 2 out]
                n192 = case shown="真" w294 {
                  frame False {
                  }
                  frame True {
                    n193 = stacked-sequence {
                      frame #0 {
                        n194 = global read "全局 1.vi" "配方编号"() -> (w300:u16)
                        n195 = call "配方.vi"() -> ("Start_Line"=w302:string[], "End_Line"=w301:string[])  [unwired: 1 in]
                        n196 = Index Array(array=w302, index=w300) -> (element=w299:string)
                        n197 = Index Array(array=w301, index=w300) -> (element=w298:string)
                        n198 = Decimal String To Number(string=w299) -> (number=w297:i32)  [unwired: 2 in, 1 out]
                        n199 = Decimal String To Number(string=w298) -> (number=w296:i32)  [unwired: 2 in, 1 out]
                        n200 = global write "全局 1.vi" "起始序号"(w297) -> ()
                        n201 = global write "全局 1.vi" "终止序号"(w296) -> ()
                      }
                      frame #1 {
                        n202 = global write "全局 1.vi" "PCTOPLC下发任务完成"(TRUE ("PCTOPLC下发任务完成")) -> ()
                      }
                    }
                  }
                }
              }
              frame #3 {
                # "允许读取配方：从PLC读取档位所在行号写入plcrecipe.csv"
                n203 = call "BuildEdgePulse.vi"("输入"=w305) -> ("上升沿"=w306:bool)  [unwired: 2 in, 2 out]
                n204 = case shown="真" w306 {
                  tunnel: w304 -> [_ w307]
                  frame False {
                  }
                  frame True {
                    n205 = stacked-sequence {
                      tunnel: w307 -> [w308 _]
                      frame #0 {
                        w309 = string[] ["N1", "1", "N1", "2", "N1", "N2", "3", "N2", "4", "N2", "N3", "5", "N3", "6", "N3", "N4", "7", "N4", "8", "N4", "N5", "9", "N5", "10"]
                        n206 = for {
                          tunnel: w309 -> [_] mode=indexing
                          tunnel: [w317] -> w315 mode=indexing
                          i -> [w318]
                          n207 = Increment(x=w318) -> (x+1=w317:i32)
                        }
                        n208 = Cluster To Array(cluster=w308) -> (array=w316:sgl[])
                        n209 = Number To Decimal String(number=w316) -> (decimal integer string=w313:string[])  [unwired: 1 in]
                        n210 = Number To Decimal String(number=w315) -> (decimal integer string=w314:string[])  [unwired: 1 in]
                        n211 = Build Array(w314, w309, w313) -> (w312:string[][])
                        n212 = Transpose 2D Array(2D array=w312) -> (transposed array=w311:string[][])
                        n213 = call "WriteCsv.vi"("相对路径"="plcrecipe.csv", "2D data"=w311) -> ()  [unwired: 2 in, 1 out]
                      }
                      frame #1 {
                        n214 = global write "全局 1.vi" "PCTOPLC读取配方完成"(TRUE ("PCTOPLC读取配方完成")) -> ()
                      }
                    }
                  }
                }
              }
              frame #4 {
                n215 = case shown="真" w324 {
                  selector: w324 -> [_ w328]
                  tunnel: w323 -> [_ w327]
                  tunnel: w322 -> [_ w329]
                  tunnel: w321 -> [_ w326]
                  tunnel: w320 -> [_ w325]
                  frame False {
                  }
                  frame True {
                    n216 = stacked-sequence {
                      tunnel: w329 -> [_ w335]
                      tunnel: w328 -> [w331 _]
                      tunnel: w327 -> [_ w334]
                      tunnel: w326 -> [_ w333]
                      tunnel: w325 -> [_ w332]
                      frame #0 {
                        n217 = call "BuildEdgePulse.vi"("输入"=w331) -> ("上升沿"=w330:bool)  [unwired: 2 in, 2 out]
                        n218 = case shown="真" w330 {
                          frame False {
                          }
                          frame True {
                            n219 = call "初始化.vi"() -> ()  [unwired: 12 in]
                          }
                        }
                      }
                      frame #1 {
                        n220 = case shown="假" w334 {
                          tunnel: w335 -> [w338 _]
                          tunnel: w333 -> [w336 _]
                          tunnel: w332 -> [w337 _]
                          frame False {
                            # "开始采集"
                            n221 = call "转换数组簇.vi"("PLC采集值"=w338) -> ()  [unwired: 2 in]
                            n222 = case shown="真" w337 {
                              tunnel: w336 -> [_ w339]
                              frame False {
                              }
                              frame True {
                                # "换档到位"
                                n223 = global write "全局 1.vi" "当前档位"(w339) -> ()
                                n224 = Number To Decimal String(number=w339) -> (decimal integer string=w340:string)  [unwired: 1 in]
                                n225 = property on="档位目标内容" class="Str"("Value"=w340) -> ()  [unwired: 2 in, 2 out]
                              }
                            }
                          }
                          frame True {
                            # "结束采集"
                          }
                        }
                      }
                    }
                  }
                }
              }
              frame #5 {
                # "读取设定参数：将UTAC设定参数写入到PLC"
                n226 = case shown="真" w343 {
                  tunnel: w342 -> [_ w346]
                  tunnel: w341 -> [_ w344]
                  frame False {
                  }
                  frame True {
                    n227 = call "BuildEdgePulse.vi"("输入"=w346) -> ("上升沿"=w345:bool)  [unwired: 2 in, 2 out]
                    n228 = case shown="真" w345 {
                      tunnel: w344 -> [_ w347]
                      frame False {
                      }
                      frame True {
                        n229 = stacked-sequence {
                          tunnel: w347 -> [w349 _]
                          frame #0 {
                            n230 = Decrement(x=w349) -> (x-1=w348:i32)
                            n231 = call "ReadCsv.vi"("相对路径"="settingparameter.csv") -> ("all rows"=w353:string[][])  [unwired: 1 in]
                            n232 = Index Array(array=w353, index (row)=w348) -> (element=w350:string[])  [unwired: 1 in]
                            n233 = Array Size(array=w350) -> (size(s)=w351:i32)
                            n234 = Less Or Equal?(x=w349, y=w351) -> (x <= y?=w352:bool)
                            n235 = case shown="真" w352 {
                              tunnel: w350 -> [_ w356]
                              frame False {
                                n236 = global write "全局 1.vi" "PCTOPLC读配方结束"(TRUE ("PCTOPLC下发配方参数完成")) -> ()
                              }
                              frame True {
                                n237 = Decimal String To Number(string=w356) -> (number=w357:i32[])  [unwired: 2 in, 1 out]
                                n238 = global write "全局 1.vi" "UTAC设定参数"(w357) -> ()
                              }
                            }
                          }
                          frame #1 {
                            n239 = global write "全局 1.vi" "PCTOPLC下发配方参数完成"(TRUE ("PCTOPLC下发配方参数完成")) -> ()
                          }
                        }
                      }
                    }
                  }
                }
              }
              frame #6 {
                n240 = call "BuildSlaveRWr.vi"() -> ("RWr"=w360:i16[][])  [unwired: 1 in]
                n241 = call "BuildRX.vi"() -> ("RX"=w359:bool[][])  [unwired: 6 in]
              }
            }
            n242 = call "BuildResPDU.vi"("从站IP"=w243, "Node RX"=w240, "Node RWr"=w241, "占用站数"=w244, "主站信息"=w252) -> ("输出字符串"=w249:string, "主站IP"=w245:u32)  [unwired: 5 in]
            n243 = UDP Write(address=w245, port or service name=w242, connection ID=w248, data in=w249, 8:w246, 9:w247) -> (error out=w251:errorcluster, 3:w250:refnum<k16>)
          }
          frame Error {
            n244 = Unbundle By Name(w363) -> ("code"=w364:i32)
            n245 = case shown="默认" w364 {
              tunnel: w363 -> [w365 _]
              tunnel: [w365 errorcluster {"status"=FALSE, "code"=0, "source"=""} ("error IO")] -> w362
              frame Default {
              }
              frame 56 {
              }
            }
          }
        }
        n246 = global read "全局 1.vi" "Exit"() -> (w217:bool)
        n247 = Wait (ms)(milliseconds to wait=u32 8 ("等待时间（毫秒）")) -> ()  [unwired: 1 out]
      }
      n248 = while {
        tunnel: [w133] -> w56
        stop <- w133 stop-if-true
        n249 = flat-sequence {
          frame #0 {
            # "显示曲线"
            n250 = call "显示曲线.vi"() -> ("曲线数组"=→"XY图":cluster{i32[], sgl[]}[])  [unwired: 2 in]
          }
        }
        n251 = event shown="[2] \"编辑配方\": 值改变" {
          selector: _ -> [_ _ _ _ _ _ _ _ _]
          dyn-events: _ -> [_ _ _ _ _ _ _ _ _]
          timeout: 100 -> [_ _ _ _ _ _ _ _ _]
          tunnel: [_ w136 _ _ _ _ _ _ _] -> w133
          event Timeout {
            n252 = event-data() -> ()  [unwired: 1 in, 3 out]
          }
          event "退出": Value Change {
            n253 = event-data() -> ()  [unwired: 1 in, 1 out]
            n254 = Two Button Dialog(message="确定退出！" ("消息"), 1:"取消" ("F按钮名称（“取消”）"), 2:"确定" ("T按钮名称（“确定”）")) -> (T button?=w137:bool)
            n255 = case shown="真" w137 {
              tunnel: [FALSE TRUE] -> w136
              frame False {
              }
              frame True {
              }
            }
            n256 = global write "全局 1.vi" "Exit"(w136) -> ()
          }
          event "编辑配方": Value Change {
            w146 = FALSE ("结束前等待")
            n257 = event-data() -> ()  [unwired: 1 in, 6 out]
            n258 = vi-ref "编辑配方.vi"() -> (w147:refnum<vi>)
            n259 = invoke class="VI" method="Run VI"(reference=w147, "Wait until done"=w146, "Auto Dispose Ref"=w146) -> (reference out=w145:refnum<vi>)  [unwired: 2 in, 4 out]
            n260 = invoke class="VI" method="FP.Open"(reference=w145) -> (reference out=w144:refnum<vi>, error out=w143:errorcluster)  [unwired: 4 in, 3 out]
            n261 = Close Reference(reference=w144, error in (no error)=w143) -> ()  [unwired: 1 out]
          }
          event "设置": Value Change {
            n262 = event-data() -> ()  [unwired: 1 in, 1 out]
            n263 = local read "总测试次数文本"() -> (w149:string)
            n264 = local read "项目编号文本"() -> (w155:string)
            n265 = local read "零件名称文本"() -> (w154:string)
            n266 = local read "零件编号文本"() -> (w153:string)
            n267 = local read "样品编号文本"() -> (w152:string)
            n268 = local read "动作数量文本"() -> (w150:string)
            n269 = local read "备注文本"() -> (w151:string)
            n270 = Decimal String To Number(string=w149) -> (number=w148:i32)  [unwired: 2 in, 1 out]
            n271 = global write "全局 1.vi" "项目编号"(w155) -> ()
            n272 = global write "全局 1.vi" "零件名称"(w154) -> ()
            n273 = global write "全局 1.vi" "零件编号"(w153) -> ()
            n274 = global write "全局 1.vi" "样品编号"(w152) -> ()
            n275 = global write "全局 1.vi" "备注"(w151) -> ()
            n276 = global write "全局 1.vi" "动作数量"(w150) -> ()
            n277 = global write "全局 1.vi" "总测试次数"(w148) -> ()
            n278 = call "WriteIni.vi"() -> ()  [unwired: 2 in]
          }
          event "档位目标内容本地": Value Change {
            n279 = event-data() -> ("NewVal"=w157:string)  [unwired: 1 in]
            n280 = Decimal String To Number(string=w157) -> (number=w156:i32)  [unwired: 2 in, 1 out]
            n281 = global write "全局 1.vi" "配方编号"(w156) -> ()
          }
          event "编辑设定参数": Value Change {
            w162 = FALSE ("结束前等待")
            n282 = event-data() -> ()  [unwired: 1 in, 6 out]
            n283 = vi-ref "编辑设定参数.vi"() -> (w159:refnum<vi>)
            n284 = invoke class="VI" method="Run VI"(reference=w159, "Wait until done"=w162, "Auto Dispose Ref"=w162) -> (reference out=w161:refnum<vi>, error out=w160:errorcluster)  [unwired: 2 in, 3 out]
            n285 = invoke class="VI" method="FP.Open"(reference=w161, error in=w160) -> (reference out=w158:refnum<vi>, error out=w163:errorcluster)  [unwired: 3 in, 3 out]
            n286 = Close Reference(reference=w158, error in (no error)=w163) -> ()  [unwired: 1 out]
          }
          event "中英文": Value Change {
            n287 = event-data() -> ("NewVal"=w164:string)  [unwired: 1 in]
            n288 = stacked-sequence {
              tunnel: w164 -> [w165 _ _ _ _ _ _ _]
              frame #0 {
                n289 = call "中英文.vi"("中英文"=w165) -> ()  [unwired: 2 in]
              }
              frame #1 {
                n290 = global read "全局 1.vi" "C-N项目信息"() -> (w175:string[])
                n291 = Index Array(array=w175) -> (element #1=w174:string, element #2=w173:string, element #3=w172:string, element #4=w171:string, element #5=w170:string, element #6=w169:string, element #7=w168:string, element #8=w167:string, element #9=w166:string)  [unwired: 9 in]
                n292 = property on="项目信息" class="Str"("Text.Text"=w174) -> ()  [unwired: 2 in, 2 out]
                n293 = property on="项目编号" class="Str"("Text.Text"=w173) -> ()  [unwired: 2 in, 2 out]
                n294 = property on="零件名称" class="Str"("Text.Text"=w172) -> ()  [unwired: 2 in, 2 out]
                n295 = property on="零件编号" class="Str"("Text.Text"=w171) -> ()  [unwired: 2 in, 2 out]
                n296 = property on="样品编号" class="Str"("Text.Text"=w170) -> ()  [unwired: 2 in, 2 out]
                n297 = property on="备注" class="Str"("Text.Text"=w169) -> ()  [unwired: 2 in, 2 out]
                n298 = property on="动作数量" class="Str"("Text.Text"=w168) -> ()  [unwired: 2 in, 2 out]
                n299 = property on="总测试次数" class="Str"("Text.Text"=w167) -> ()  [unwired: 2 in, 2 out]
                n300 = property on="设置" class="Bool"("BoolText.Text"=w166) -> ()  [unwired: 2 in, 2 out]
              }
              frame #2 {
                n301 = global read "全局 1.vi" "C-NDO信号"() -> (w182:string[])
                n302 = Index Array(array=w182) -> (element #1=w181:string, element #2=w180:string, element #3=w179:string, element #4=w178:string, element #5=w177:string, element #6=w176:string)  [unwired: 6 in]
                n303 = property on="UTACTOPC的DO信号" class="Str"("Text.Text"=w181) -> ()  [unwired: 2 in, 2 out]
                n304 = property on="UTAC运行/停机" class="Bool (严格)"("BoolText.Text"=w180) -> ()  [unwired: 2 in, 2 out]
                n305 = property on="UTAC故障" class="Bool (严格)"("BoolText.Text"=w179) -> ()  [unwired: 2 in, 2 out]
                n306 = property on="UTAC故障复位" class="Bool (严格)"("BoolText.Text"=w178) -> ()  [unwired: 2 in, 2 out]
                n307 = property on="UTAC急停" class="Bool (严格)"("BoolText.Text"=w177) -> ()  [unwired: 2 in, 2 out]
                n308 = property on="UTAC复位到原点" class="Bool (严格)"("BoolText.Text"=w176) -> ()  [unwired: 2 in, 2 out]
              }
              frame #3 {
                n309 = global read "全局 1.vi" "C-NDI信号"() -> (w191:string[])
                n310 = Index Array(array=w191) -> (element #1=w190:string, element #2=w189:string, element #3=w188:string, element #4=w187:string, element #5=w186:string, element #6=w185:string, element #7=w184:string, element #8=w183:string)  [unwired: 8 in]
                n311 = property on="PCOUTAC的DI信号" class="Str"("Text.Text"=w190) -> ()  [unwired: 2 in, 2 out]
                n312 = property on="PC运行/停机" class="Bool (严格)"("BoolText.Text"=w189) -> ()  [unwired: 2 in, 2 out]
                n313 = property on="PC故障" class="Bool (严格)"("BoolText.Text"=w188) -> ()  [unwired: 2 in, 2 out]
                n314 = property on="PC学习" class="Bool (严格)"("BoolText.Text"=w187) -> ()  [unwired: 2 in, 2 out]
                n315 = property on="PC急停" class="Bool (严格)"("BoolText.Text"=w186) -> ()  [unwired: 2 in, 2 out]
                n316 = property on="PC正在换挡" class="Bool (严格)"("BoolText.Text"=w185) -> ()  [unwired: 2 in, 2 out]
                n317 = property on="PC换挡到位" class="Bool (严格)"("BoolText.Text"=w184) -> ()  [unwired: 2 in, 2 out]
                n318 = property on="PC换挡不成功" class="Bool (严格)"("BoolText.Text"=w183) -> ()  [unwired: 2 in, 2 out]
              }
              frame #4 {
                n319 = global read "全局 1.vi" "C-N设置"() -> (w196:string[])
                n320 = Index Array(array=w196) -> (element #1=w195:string, element #2=w194:string, element #3=w193:string, element #4=w192:string)  [unwired: 4 in]
                n321 = property on="设置" class="Str"("Text.Text"=w195) -> ()  [unwired: 2 in, 2 out]
                n322 = property on="退出" class="Bool"("BoolText.Text"=w194) -> ()  [unwired: 2 in, 2 out]
                n323 = property on="编辑配方" class="Bool"("BoolText.Text"=w193) -> ()  [unwired: 2 in, 2 out]
                n324 = property on="编辑设定参数" class="Bool"("BoolText.Text"=w192) -> ()  [unwired: 2 in, 2 out]
              }
              frame #5 {
                n325 = global read "全局 1.vi" "C-N目标档位"() -> (w199:string[])
                n326 = Index Array(array=w199) -> (element #1=w198:string, element #2=w197:string)  [unwired: 2 in]
                n327 = property on="UTACTOPC的目标档位" class="Str"("Text.Text"=w198) -> ()  [unwired: 2 in, 2 out]
                n328 = property on="档位目标" class="Str"("Text.Text"=w197) -> ()  [unwired: 2 in, 2 out]
              }
              frame #6 {
                n329 = global read "全局 1.vi" "C-N当前档位"() -> (w202:string[])
                n330 = Index Array(array=w202) -> (element #1=w201:string, element #2=w200:string)  [unwired: 2 in]
                n331 = property on="PCTOUTAC的当前档位" class="Str"("Text.Text"=w201) -> ()  [unwired: 2 in, 2 out]
                n332 = property on="当前档位" class="Str"("Text.Text"=w200) -> ()  [unwired: 2 in, 2 out]
              }
              frame #7 {
                n333 = global read "全局 1.vi" "C-N远程/本地"() -> (w205:string[])
                n334 = Index Array(array=w205) -> (element #1=w204:string, element #2=w203:string)  [unwired: 2 in]
                n335 = property on="远程/本地控制标题" class="Str"("Text.Text"=w204) -> ()  [unwired: 2 in, 2 out]
                n336 = property on="远程/本地控制" class="Bool (严格)"("BoolText.Text"=w203) -> ()  [unwired: 2 in, 2 out]
              }
            }
          }
          event "PC启动信号": Value Change {
            n337 = event-data() -> ()  [unwired: 1 in, 6 out]
            n338 = global write "全局 1.vi" "PCTOPLC发送启动信号"(TRUE ("PCTOPLC发送启动信号")) -> ()
          }
          event "擦除曲线": Value Change {
            # "初始化"
            n339 = event-data() -> ()  [unwired: 1 in, 6 out]
            n340 = call "初始化.vi"() -> ()  [unwired: 12 in]
          }
        }
      }
    }
  }
  n341 = And(x=w3, y=TRUE) -> (x .and. y?=w1:bool)
  n342 = UDP Close(connection ID=w5, 8:w4) -> ()  [unwired: 2 out]
  n343 = case shown="真" w1 {
    frame False {
    }
    frame True {
      n344 = invoke class="VI" method="FP.Close"() -> (reference out=w368:refnum<vi>, error out=w367:errorcluster)  [unwired: 3 in, 1 out]
      n345 = Close Reference(reference=w368, error in (no error)=w367) -> ()  [unwired: 1 out]
    }
  }
